vi "CreateList.vi"(9 "Range":dbl, 10 "Increment (V)":dbl=0.5 min=0.0 max=63.0, 11 "Style":u16(ring) items=["Ramp+-", "Pos-Neg", "Ramp", "0 Ramp", "Double+-"]) -> (3 "Ramp Pattern":dbl[](array[numeric]))   [LabVIEW 2019, in "2231A.lvclass"]
uses:
  2231A.lvclass
  <vilib>/Analysis/1siggen.llb/Ramp Pattern by Delta.vi
  <vilib>/Analysis/NI_AALBase.lvlib
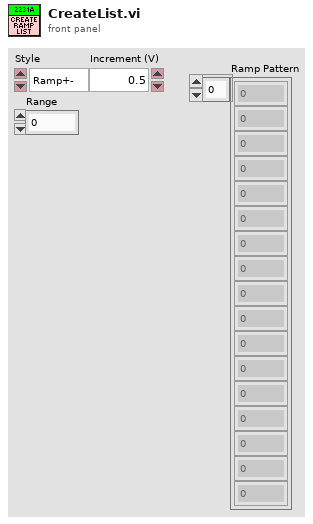
[diagram p1: front panel]
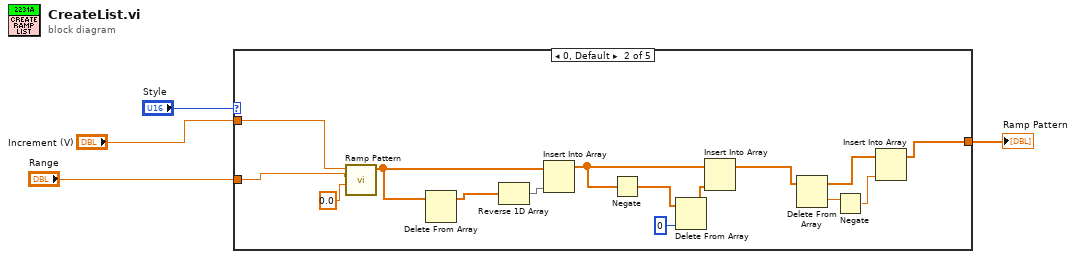
[diagram p0: block diagram]
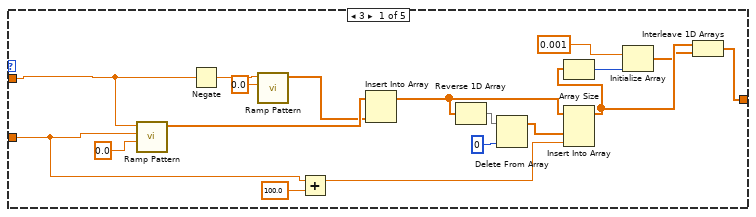
[diagram p2: hidden frame]
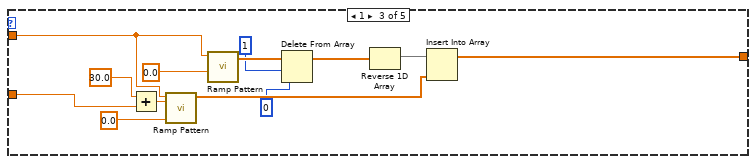
[diagram p3: hidden frame]
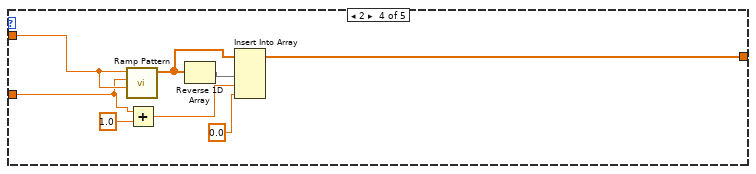
[diagram p4: hidden frame]
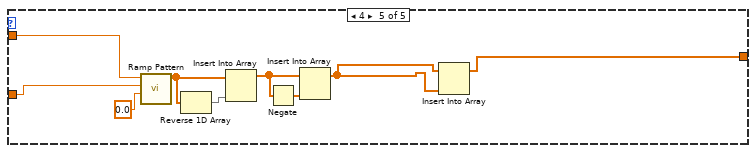
[diagram p5: hidden frame]
diagram:
  n1 = case shown="0, Default" "Style" {
    tunnel: [w7 w23 w46 w56 w59] -> w4
    tunnel: "Increment (V)" -> [w9 w37 w39 w55 w62]
    tunnel: "Range" -> [w5 w33 w38 w51 w61]
    frame 3 {
      n2 = call-poly <vilib>:"Ramp Pattern.vi"("start"=0.0, "end"=w5, "delta"=w9) -> ("Ramp Pattern"=w19:dbl[])  [unwired: 6 in, 2 out]
      n3 = Negate(x=w9) -> (-x=w17:dbl)
      n4 = call-poly <vilib>:"Ramp Pattern.vi"("end"=0.0, "delta"=w17) -> ("Ramp Pattern"=w18:dbl[])  [unwired: 7 in, 2 out]
      n5 = Add(x=w5, y=100.0) -> (x+y=w11:dbl)
      n6 = Insert Into Array(array=w19, new element=w18) -> (w14:dbl[])  [unwired: 1 in]
      n7 = Reverse 1D Array(array=w14) -> (reversed array=w13:dbl[])
      n8 = Delete From Array(array=w13, index=0) -> (array with subset deleted=w12:dbl[])  [unwired: 1 in, 1 out]
      n9 = Insert Into Array(array=w14, new element #1=w12, new element #2=w11) -> (w8:dbl[])  [unwired: 1 in]
      n10 = Array Size(array=w8) -> (size(s)=w22:i32)
      n11 = Initialize Array(0.001 ("element"), w22) -> (w6:dbl[])
      n12 = Interleave 1D Arrays(w8, w6) -> (w7:dbl[])
    }
    frame 0, Default {
      n13 = call-poly <vilib>:"Ramp Pattern.vi"("start"=0.0, "end"=w33, "delta"=w37) -> ("Ramp Pattern"=w32:dbl[])  [unwired: 6 in, 2 out]
      n14 = Delete From Array(array=w32) -> (array with subset deleted=w31:dbl[])  [unwired: 2 in, 1 out]
      n15 = Reverse 1D Array(array=w31) -> (reversed array=w36:dbl[])
      n16 = Insert Into Array(array=w32, new element=w36) -> (w35:dbl[])  [unwired: 1 in]
      n17 = Negate(x=w35) -> (-x=w30:dbl[])
      n18 = Delete From Array(array=w30, index=0) -> (array with subset deleted=w28:dbl[])  [unwired: 1 in, 1 out]
      n19 = Insert Into Array(array=w35, new element=w28) -> (w27:dbl[])  [unwired: 1 in]
      n20 = Delete From Array(array=w27) -> (deleted portion=w26:dbl, array with subset deleted=w24:dbl[])  [unwired: 2 in]
      n21 = Negate(x=w26) -> (-x=w25:dbl)
      n22 = Insert Into Array(array=w24, new element=w25) -> (w23:dbl[])  [unwired: 1 in]
    }
    frame 1 {
      n23 = Add(x=30.0, y=w38) -> (x+y=w50:dbl)
      n24 = call-poly <vilib>:"Ramp Pattern.vi"("start"=0.0, "end"=w50, "delta"=w39) -> ("Ramp Pattern"=w47:dbl[])  [unwired: 6 in, 2 out]
      n25 = call-poly <vilib>:"Ramp Pattern.vi"("start"=0.0, "delta"=w39) -> ("Ramp Pattern"=w49:dbl[])  [unwired: 7 in, 2 out]
      n26 = Delete From Array(array=w49, length=1, index=0) -> (array with subset deleted=w43:dbl[])  [unwired: 1 out]
      n27 = Reverse 1D Array(array=w43) -> (reversed array=w48:dbl[])
      n28 = Insert Into Array(array=w48, new element=w47) -> (w46:dbl[])  [unwired: 1 in]
    }
    frame 2 {
      n29 = call-poly <vilib>:"Ramp Pattern.vi"("start"=w55, "end"=w51, "delta"=w55) -> ("Ramp Pattern"=w58:dbl[])  [unwired: 6 in, 2 out]
      n30 = Add(x=w51, y=1.0) -> (x+y=w52:dbl)
      n31 = Reverse 1D Array(array=w58) -> (reversed array=w57:dbl[])
      n32 = Insert Into Array(array=w58, new element #1=w57, new element #2=w52, new element #3=0.0 ("new element/subarray")) -> (w56:dbl[])  [unwired: 1 in]
    }
    frame 4 {
      n33 = call-poly <vilib>:"Ramp Pattern.vi"("start"=0.0, "end"=w61, "delta"=w62) -> ("Ramp Pattern"=w67:dbl[])  [unwired: 6 in, 2 out]
      n34 = Reverse 1D Array(array=w67) -> (reversed array=w66:dbl[])
      n35 = Insert Into Array(array=w67, new element=w66) -> (w65:dbl[])  [unwired: 1 in]
      n36 = Negate(x=w65) -> (-x=w64:dbl[])
      n37 = Insert Into Array(array=w65, new element=w64) -> (w60:dbl[])  [unwired: 1 in]
      n38 = Insert Into Array(array=w60, new element=w60) -> (w59:dbl[])  [unwired: 1 in]
    }
  }
  "Ramp Pattern" <- w4
